vi "周期设置_总磷总氮.vi"() -> ()   [LabVIEW 2016, in "斯坦道总磷总氮.lvlib"]
uses:
  <vilib>/Utility/miscctls.llb/LVPointTypeDef.ctl
  <vilib>/Utility/config.llb/NI_LVConfig.lvlib
panel:
  in  "运行周期":T1={"运行模式"=enum."维护模式", "质控频次"=enum."关闭", "空白核查时间"=2, "跨度核查时间"=6, "24H周期设置"=[]} {"跨度核查时间" items=["00H", "01H", "02H", "03H", "04H", "05H", "06H", "07H", "08H", "09H", "10H", "11H", "12H", "13H", "14H", "15H", "16H", "17H", "18H", "19H", "20H", "21H", "22H", "23H", "关闭"]; "空白核查时间" items=["00H", "01H", "02H", "03H", "04H", "05H", "06H", "07H", "08H", "09H", "10H", "11H", "12H", "13H", "14H", "15H", "16H", "17H", "18H", "19H", "20H", "21H", "22H", "23H", "关闭"]}
  # "运行模式："
  # "质控频次："
  # "空白核查时间："
  # "跨度核查时间："
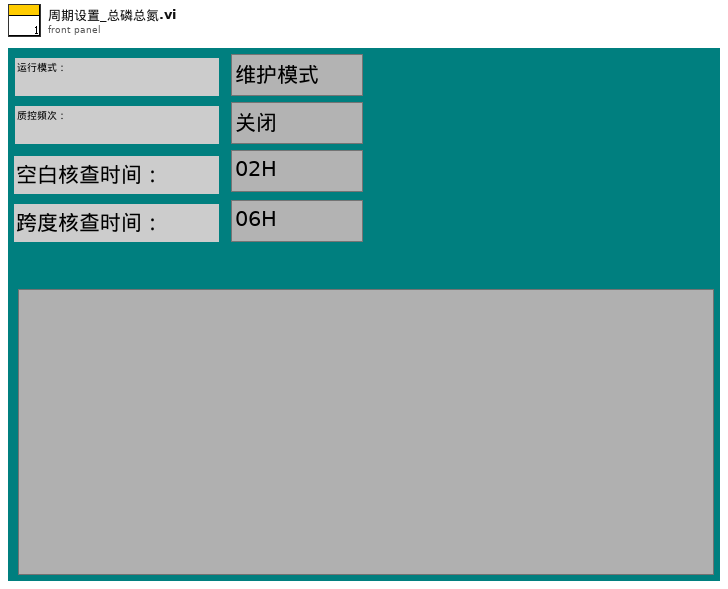
[diagram p1: front panel]
types:
  T1 = cluster{"运行模式":enum16{"维护模式", "常规模式", "应急模式", "质控模式"}, "质控频次":enum16{"关闭", "每天", "星期一", "星期二", "星期三", "星期四", "星期五", "星期六", "星期日"}, "空白核查时间":u16, "跨度核查时间":u16, "24H周期设置":bool[]}
  T2 = typedef "LVPointTypeDef.ctl" = cluster{"Horizontal":i16, "Vertical":i16}
  T3 = cluster{"站号":u16, "量程切换":enum32{"H", "L", "AUTO"}, "控制命令":enum16{"启动测量", "标样核查", "零点核查", "跨度核查", "空白测试", "平行样测试", "加标回收", "空白校准", "标样校准", "初始化（清洗）", "停止测试", "仪器重启", "校时", "模式设置", "测量间隔设置"}, "模式设置":enum16{"待机", "连续模式", "周期模式", "定点模式", "受控模式", "手动模式"}, "测量间隔":u16}
  T4 = enum16{"启动测量", "标样核查", "零点核查", "跨度核查", "空白测试", "平行样测试", "加标回收", "空白校准", "标样校准", "初始化（清洗）", "停止测试", "仪器重启", "校时", "模式设置", "测量间隔设置"}
  T5 = enum16{"关闭", "每天", "星期一", "星期二", "星期三", "星期四", "星期五", "星期六", "星期日"}
  T6 = typedef "LVDateTimeRec.ctl" = cluster{"秒数的小数部分":dbl, "秒":i32, "分":i32, "时":i32, "日":i32, "月":i32, "年":i32, "天数（周）":i32, "天数（年）":i32, "DST":i32}
  T7 = enum32{"Bad", "Idle", "Run top level", "Running"}
  T8 = cluster{"水样测试量程模式":enum16{"H", "L", "AUTO"}, "空白核查量程模式":enum16{"H", "L", "AUTO"}, "跨度核查量程模式":enum16{"H", "L", "AUTO"}}
  T9 = typedef "NI_LVConfig.lvlib/Config Data RefNum.ctl" = refnum<k1>
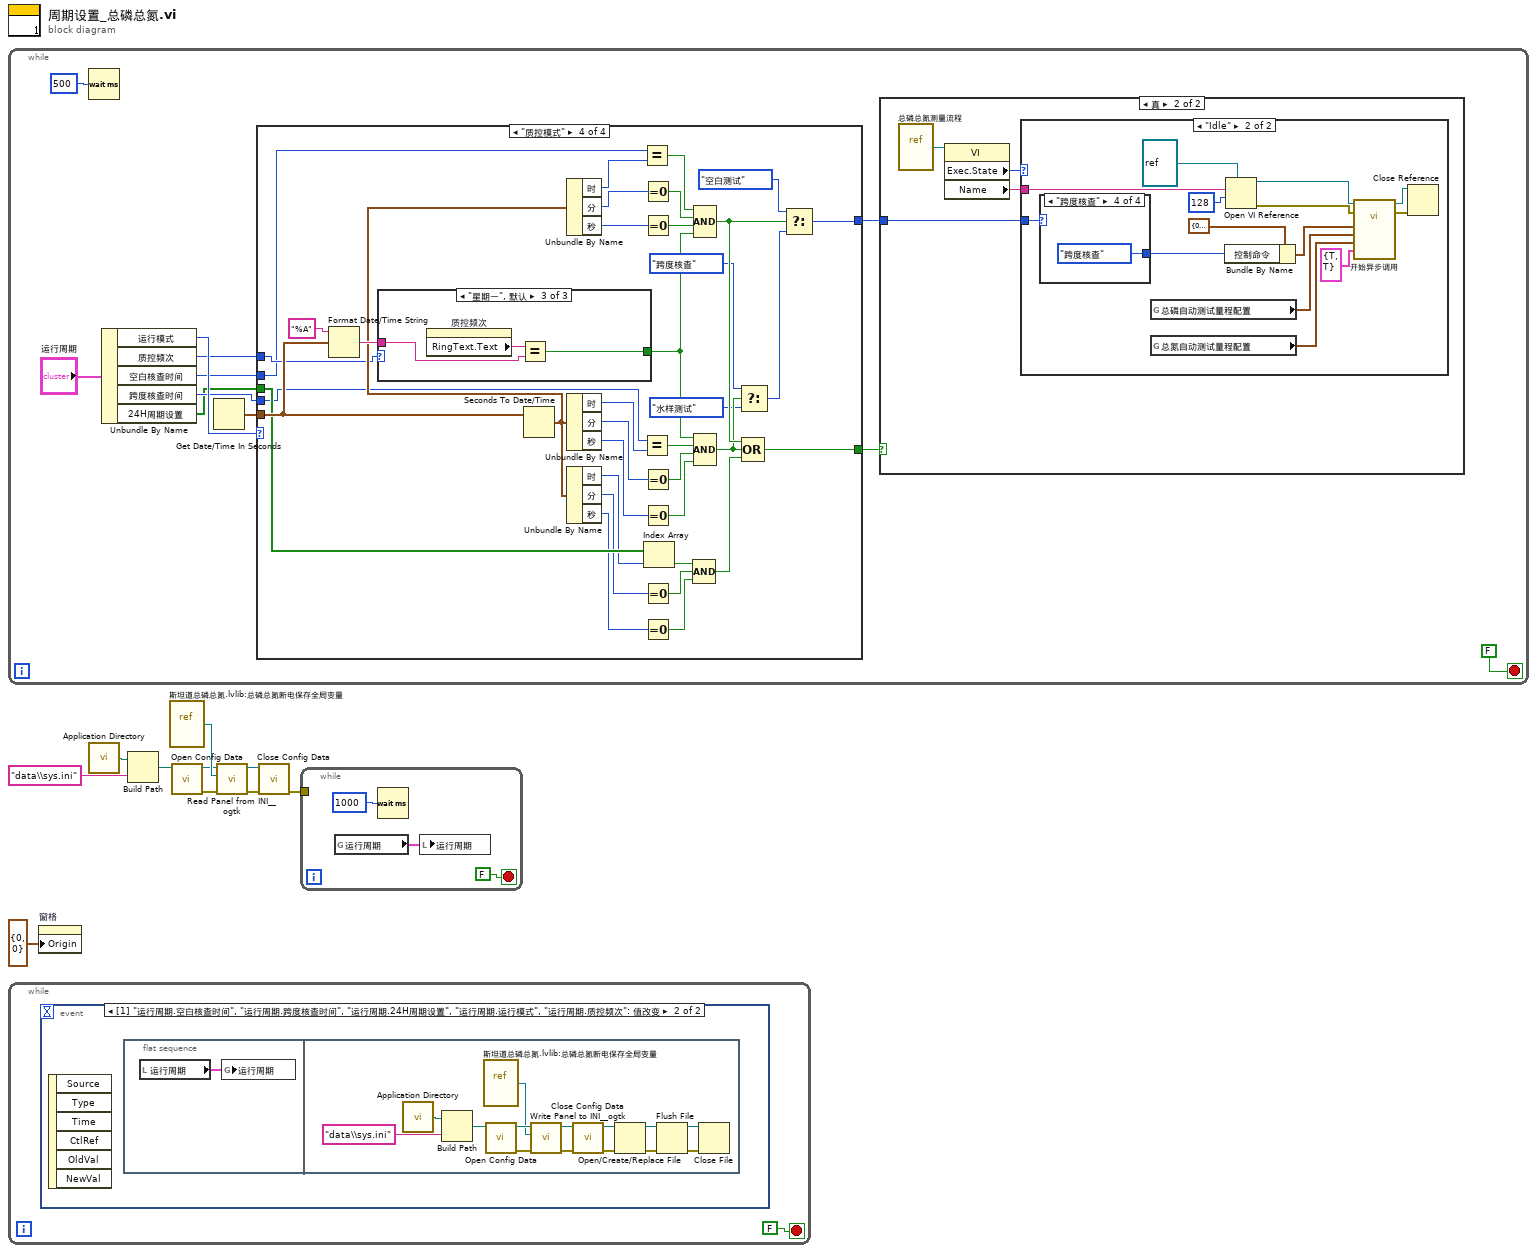
[diagram p0: block diagram]
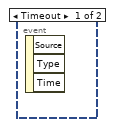
[diagram p2: hidden frame]
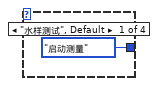
[diagram p5: hidden frame]
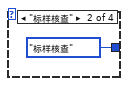
[diagram p6: hidden frame]
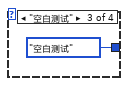
[diagram p7: hidden frame]
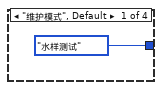
[diagram p8: hidden frame]
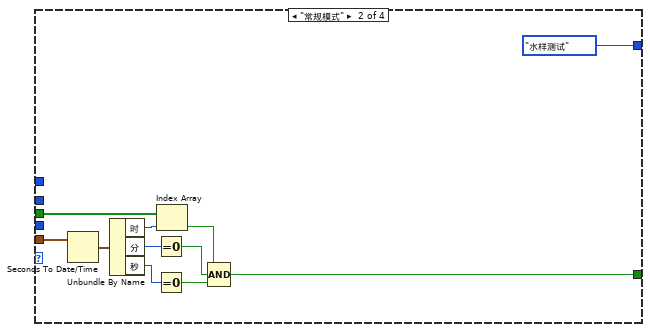
[diagram p9: hidden frame]
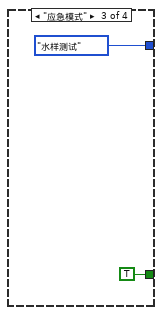
[diagram p10: hidden frame]
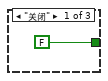
[diagram p11: hidden frame]
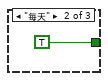
[diagram p12: hidden frame]
diagram:
  n1 = while {
    stop <- FALSE stop-if-true
    n2 = Wait (ms)(milliseconds to wait=u32 500 ("等待时间（毫秒）")) -> ()  [unwired: 1 out]
    n3 = Unbundle By Name("运行周期") -> ("运行模式"=w17:enum16{"维护模式", "常规模式", "应急模式", "质控模式"}, "质控频次"=w16:T5, "空白核查时间"=w15:u16, "跨度核查时间"=w14:u16, "24H周期设置"=w13:bool[])
    n4 = Get Date/Time In Seconds() -> (seconds since 1Jan1904=w21:timestamp)
    n5 = case shown="\"质控模式\"" w17 {
      tunnel: w21 -> [_ w54 _ w93]
      tunnel: w13 -> [_ w51 _ w90]
      tunnel: [_ w45 TRUE w70] -> w12
      tunnel: [enum16{"水样测试", "标样核查", "空白测试", "跨度核查"}."水样测试" ("仪器测试类型") enum16{"水样测试", "标样核查", "空白测试", "跨度核查"}."水样测试" ("仪器测试类型") enum16{"水样测试", "标样核查", "空白测试", "跨度核查"}."水样测试" ("仪器测试类型") w63] -> w11
      tunnel: w16 -> [_ _ _ w60]
      tunnel: w15 -> [_ _ _ w59]
      tunnel: w14 -> [_ _ _ w58]
      frame "维护模式", Default {
      }
      frame "常规模式" {
        n6 = Seconds To Date/Time(time stamp (now)=w54) -> (date time rec=w53:T6)  [unwired: 1 in]
        n7 = Unbundle By Name(w53) -> ("时"=w52:i32, "分"=w50:i32, "秒"=w49:i32)
        n8 = Equal To 0?(x=w50) -> (x = 0?=w47:bool)
        n9 = Equal To 0?(x=w49) -> (x = 0?=w46:bool)
        n10 = Index Array(array=w51, index=w52) -> (element=w48:bool)
        n11 = Compound Arithmetic op=AND ("复合运算")(w48, w47, w46) -> (w45:bool)
      }
      frame "应急模式" {
      }
      frame "质控模式" {
        n12 = Format Date/Time String(time format string (%c)="%A" ("时间格式字符串(%c)"), seconds (now)=w93) -> (date/time string=w91:string)  [unwired: 1 in]
        n13 = case shown="\"星期一\", 默认" w60 {
          tunnel: w91 -> [_ _ w97]
          tunnel: [FALSE TRUE w96] -> w61
          frame "关闭" {
          }
          frame "每天" {
          }
          frame "星期一", Default {
            n14 = property on="质控频次" class="Enum (严格)"() -> ("RingText.Text"=w98:string)  [unwired: 2 in, 2 out]
            n15 = Equal?(x=w98, y=w97) -> (x = y?=w96:bool)
          }
        }
        n16 = Seconds To Date/Time(time stamp (now)=w93) -> (date time rec=w74:T6)  [unwired: 1 in]
        n17 = Unbundle By Name(w74) -> ("时"=w83:i32, "分"=w82:i32, "秒"=w81:i32)
        n18 = Unbundle By Name(w74) -> ("时"=w75:i32, "分"=w76:i32, "秒"=w77:i32)
        n19 = Unbundle By Name(w74) -> ("时"=w89:i32, "分"=w87:i32, "秒"=w85:i32)
        n20 = Equal?(x=w59, y=w83) -> (x = y?=w80:bool)
        n21 = Equal?(x=w58, y=w75) -> (x = y?=w73:bool)
        n22 = Equal To 0?(x=w82) -> (x = 0?=w79:bool)
        n23 = Equal To 0?(x=w81) -> (x = 0?=w78:bool)
        n24 = Equal To 0?(x=w76) -> (x = 0?=w72:bool)
        n25 = Equal To 0?(x=w77) -> (x = 0?=w71:bool)
        n26 = Equal To 0?(x=w87) -> (x = 0?=w86:bool)
        n27 = Equal To 0?(x=w85) -> (x = 0?=w84:bool)
        n28 = Index Array(array=w90, index=w89) -> (element=w88:bool)
        n29 = Compound Arithmetic op=AND ("复合运算")(w88, w86, w84) -> (w62:bool)
        n30 = Compound Arithmetic op=AND ("复合运算")(w80, w79, w78, w61) -> (w69:bool)
        n31 = Compound Arithmetic op=AND ("复合运算")(w61, w73, w72, w71) -> (w67:bool)
        n32 = Select(t=enum16{"水样测试", "标样核查", "空白测试", "跨度核查"}."跨度核查" ("仪器测试类型"), s=w67, f=enum16{"水样测试", "标样核查", "空白测试", "跨度核查"}."水样测试" ("仪器测试类型")) -> (s? t:f=w65:enum16{"水样测试", "标样核查", "空白测试", "跨度核查"})
        n33 = Compound Arithmetic op=OR ("复合运算")(w69, w67, w62) -> (w70:bool)
        n34 = Select(t=enum16{"水样测试", "标样核查", "空白测试", "跨度核查"}."空白测试" ("仪器测试类型"), s=w69, f=w65) -> (s? t:f=w63:enum16{"水样测试", "标样核查", "空白测试", "跨度核查"})
      }
    }
    n35 = case shown="真" w12 {
      tunnel: w11 -> [_ w23]
      frame False {
      }
      frame True {
        n36 = vi-ref "总磷总氮测量流程.vi"() -> (w24:refnum<vi>)
        n37 = property class="VI"(reference=w24) -> ("Exec.State"=w22:T7, "Name"=w25:string)  [unwired: 1 in, 2 out]
        n38 = case shown="\"Idle\"" w22 {
          tunnel: w25 -> [_ w35]
          tunnel: w23 -> [_ w26]
          frame "Bad", Default {
          }
          frame "Idle" {
            n39 = case shown="\"跨度核查\"" w26 {
              tunnel: [T4."启动测量" ("控制命令") T4."标样核查" ("控制命令") T4."空白测试" ("控制命令") T4."跨度核查" ("控制命令")] -> w31
              frame "水样测试", Default {
              }
              frame "标样核查" {
              }
              frame "空白测试" {
              }
              frame "跨度核查" {
              }
            }
            n40 = global read "总磷总氮断电保存全局变量.vi" "总磷自动测试量程配置"() -> (w30:T8)
            n41 = global read "总磷总氮断电保存全局变量.vi" "总氮自动测试量程配置"() -> (w29:T8)
            n42 = Bundle By Name(cluster=T3 {"站号"=0, "量程切换"=enum."H", "控制命令"=enum."启动测量", "模式设置"=enum."待机", "测量间隔"=0} ("参数"), "控制命令"=w31) -> (w32:T3)
            n43 = Open VI Reference(type specifier VI Refnum (for type only)=refnum<vi> refnum, vi path=w35, options=128 ("选项")) -> (vi reference=w36:refnum<vi>, error out=w37:errorcluster)  [unwired: 3 in]
            n44 = call-by-ref "开始异步调用"(reference=w36, error in=w37, "启动参数"=cluster{"总磷":bool, "总氮":bool} {"总磷"=TRUE, "总氮"=TRUE}, "总氮量程模式"=w29, "总磷量程模式"=w30, "参数"=w32) -> (reference out=w38:refnum<vi>, error out=w39:errorcluster)  [unwired: 8 in]
            n45 = Close Reference(reference=w38, error in (no error)=w39) -> ()  [unwired: 1 out]
          }
        }
      }
    }
  }
  n46 = while {
    stop <- FALSE stop-if-true
    n47 = event shown="[1] \"运行周期.空白核查时间\", \"运行周期.跨度核查时间\", \"运行周期.24H周期设置\", \"运行周期.运行模式\", \"运行周期.质控频次\": 值改变" {
      selector: _ -> [_ _]
      dyn-events: _ -> [_ _]
      timeout: _ -> [_ _]
      event Timeout {
        n48 = event-data() -> ()  [unwired: 1 in, 3 out]
      }
      event "运行周期.空白核查时间", "运行周期.跨度核查时间", "运行周期.24H周期设置", "运行周期.运行模式", "运行周期.质控频次": Value Change {
        n49 = event-data() -> ()  [unwired: 1 in, 6 out]
        n50 = flat-sequence {
          frame #0 {
            n51 = local read "运行周期"() -> (w100:T1)
            n52 = global write "总磷总氮断电保存全局变量.vi" "运行周期"(w100) -> ()
          }
          frame #1 {
            n53 = call <vilib>:"Application Directory.vi"() -> ("Application Directory"=w114:path)
            n54 = Build Path(base path=w114, name or relative path="data\\sys.ini" ("名称或相对路径")) -> (appended path=w112:path)
            n55 = vi-ref "斯坦道总磷总氮.lvlib:总磷总氮断电保存全局变量.vi"() -> (w110:refnum<vi>)
            n56 = call <vilib>:"Open Config Data.vi"("configuration file path"=w112) -> ("error out"=w108:errorcluster, "refnum"=w111:T9)  [unwired: 8 in, 1 out]
            n57 = call <userlib>:"Write Panel to INI__ogtk.vi"("error in (no error)"=w108, "VI ref"=w110, "refnum"=w111) -> ("error out"=w107:errorcluster, "refnum out"=w109:T9)  [unwired: 7 in]
            n58 = call <vilib>:"Close Config Data.vi"("error in (no error)"=w107, "refnum"=w109) -> ("error out"=w102:errorcluster, "file path"=w101:path)  [unwired: 8 in]
            n59 = Open/Create/Replace File(file path (use dialog)=w101, error in=w102) -> (refnum out=w105:refnum<file>, error out=w106:errorcluster)  [unwired: 4 in, 1 out]
            n60 = Flush File(refnum=w105, error in=w106) -> (refnum out=w104:refnum<file>, error out=w103:errorcluster)
            n61 = Close File(refnum=w104, error in=w103) -> ()  [unwired: 2 out]
          }
        }
      }
    }
  }
  n62 = property on="窗格" class="Pane"("Origin"=T2 {"Horizontal"=0, "Vertical"=0} ("原点")) -> ()  [unwired: 2 in, 2 out]
  n63 = call <vilib>:"Application Directory.vi"() -> ("Application Directory"=w3:path)
  n64 = Build Path(base path=w3, name or relative path="data\\sys.ini" ("名称或相对路径")) -> (appended path=w5:path)
  n65 = vi-ref "斯坦道总磷总氮.lvlib:总磷总氮断电保存全局变量.vi"() -> (w7:refnum<vi>)
  n66 = call <vilib>:"Open Config Data.vi"("configuration file path"=w5) -> ("error out"=w9:errorcluster, "refnum"=w6:T9)  [unwired: 8 in, 1 out]
  n67 = call <userlib>:"Read Panel from INI__ogtk.vi"("error in (no error)"=w9, "VI ref"=w7, "refnum"=w6) -> ("error out"=w10:errorcluster, "refnum out"=w8:T9)  [unwired: 7 in]
  n68 = call <vilib>:"Close Config Data.vi"("error in (no error)"=w10, "refnum"=w8) -> ("error out"=w2:errorcluster)  [unwired: 8 in, 1 out]
  n69 = while {
    tunnel: w2 -> [_]
    stop <- FALSE stop-if-true
    n70 = global read "总磷总氮断电保存全局变量.vi" "运行周期"() -> (w115:T1)
    n71 = Wait (ms)(milliseconds to wait=u32 1000 ("等待时间（毫秒）")) -> ()  [unwired: 1 out]
    n72 = local write "运行周期"(w115) -> ()
  }
